vi "GEOM_Adjust_Sizes.vi"(4 "remaining Y":i32, 6 "remainingX":i32, 7 "BinCorrectionType":T7(ring), 8 "Binning":T5={"x"=1, "y"=1} {"y" min=1; "x" min=1}, 9 "sections":T6[](array[typedef]), 10 "Amplifier":T1={"number"=0, "type"=0, "rotated"=0, "fliped"=0, "FPAcoord"={"xstart"=1, "ystart"=1}, "Physical_size"={"columns"=0, "rows"=0}, "predata"={"columns"=0, "rows"=0}, "postdata"={"columns"=0, "rows"=0}, "Req ROIs"=[], "Corr ROI"=[], "Detnumber"=0, "ampID"="", "discard"=0} {"fliped" items=["none", "horizontal", "vertical"]; "type" items=["LL", "LR", "UL", "UR"]}) -> (1 "binned amp":T1={"number"=0, "type"=0, "rotated"=0, "fliped"=0, "FPAcoord"={"xstart"=1, "ystart"=1}, "Physical_size"={"columns"=0, "rows"=0}, "predata"={"columns"=0, "rows"=0}, "postdata"={"columns"=0, "rows"=0}, "Req ROIs"=[], "Corr ROI"=[], "Detnumber"=0, "ampID"="", "discard"=0} {"fliped" items=["none", "horizontal", "vertical"]; "type" items=["LL", "LR", "UL", "UR"]}, 2 "non-binned amp":T1={"number"=0, "type"=0, "rotated"=0, "fliped"=0, "FPAcoord"={"xstart"=1, "ystart"=1}, "Physical_size"={"columns"=0, "rows"=0}, "predata"={"columns"=0, "rows"=0}, "postdata"={"columns"=0, "rows"=0}, "Req ROIs"=[], "Corr ROI"=[], "Detnumber"=0, "ampID"="", "discard"=0} {"fliped" items=["none", "horizontal", "vertical"]; "type" items=["LL", "LR", "UL", "UR"]})   [LabVIEW 2016]
uses:
  GEOM_Moifier.ctl
  GEOM_Amplifier.ctl
  GEOM_AmpType.ctl
  GEOM_ROI.ctl
  GEOM_Coords.ctl
  GEOM_Binning.ctl
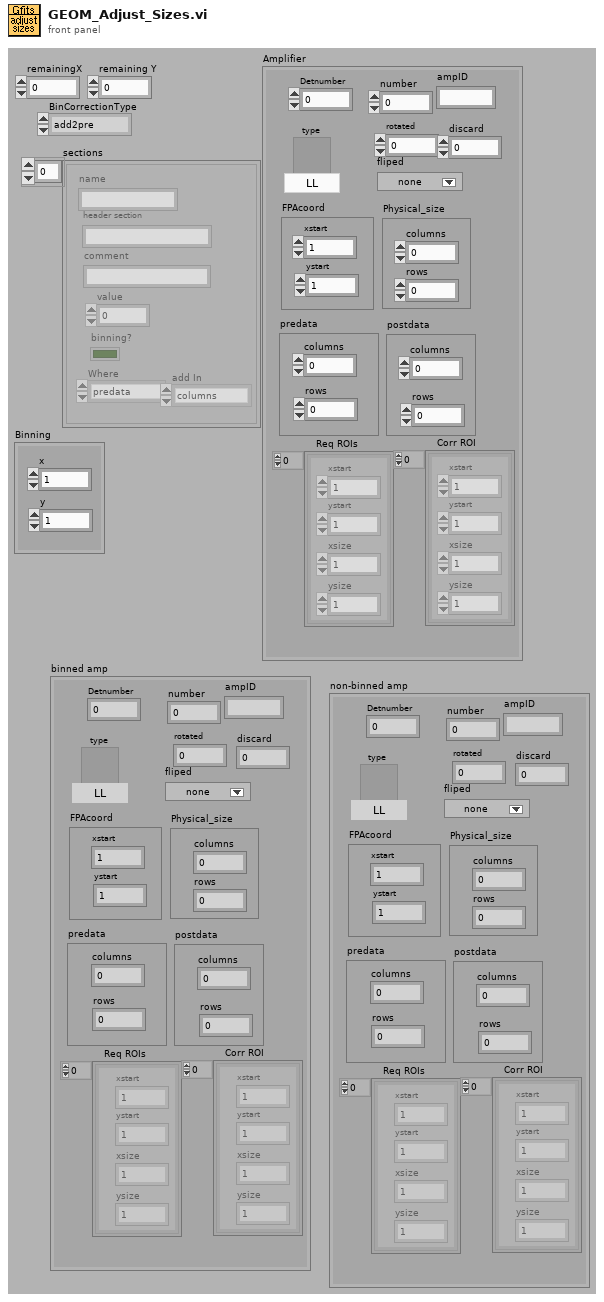
[diagram p1: front panel]
types:
  T1 = typedef "GEOM_Amplifier.ctl" = cluster{"number":i32, "type":T2, "rotated":i16, "fliped":u16, "FPAcoord":cluster{"xstart":i32, "ystart":i32}, "Physical_size":cluster{"columns":i32, "rows":i32}, "predata":cluster{"columns":i32, "rows":i32}, "postdata":cluster{"columns":i32, "rows":i32}, "Req ROIs":T3, "Corr ROI":T3, "Detnumber":i32, "ampID":string, "discard":i32}
  T2 = typedef "GEOM_AmpType.ctl" = u16
  T3 = typedef "GEOM_ROI.ctl" = T4[]
  T4 = typedef "GEOM_Coords.ctl" = cluster{"xstart":u32, "ystart":u32, "xsize":u32, "ysize":u32}
  T5 = typedef "GEOM_Binning.ctl" = cluster{"x":u32, "y":u32}
  T6 = typedef "GEOM_Moifier.ctl" = cluster{"name":string, "header section":string, "comment":string, "value":i32, "binning?":bool, "Where":enum16{"predata", "postdata"}, "add In":enum16{"columns", "rows", "none"}}
  T7 = enum16{"add2pre", "add2post", "add2data", "none"}
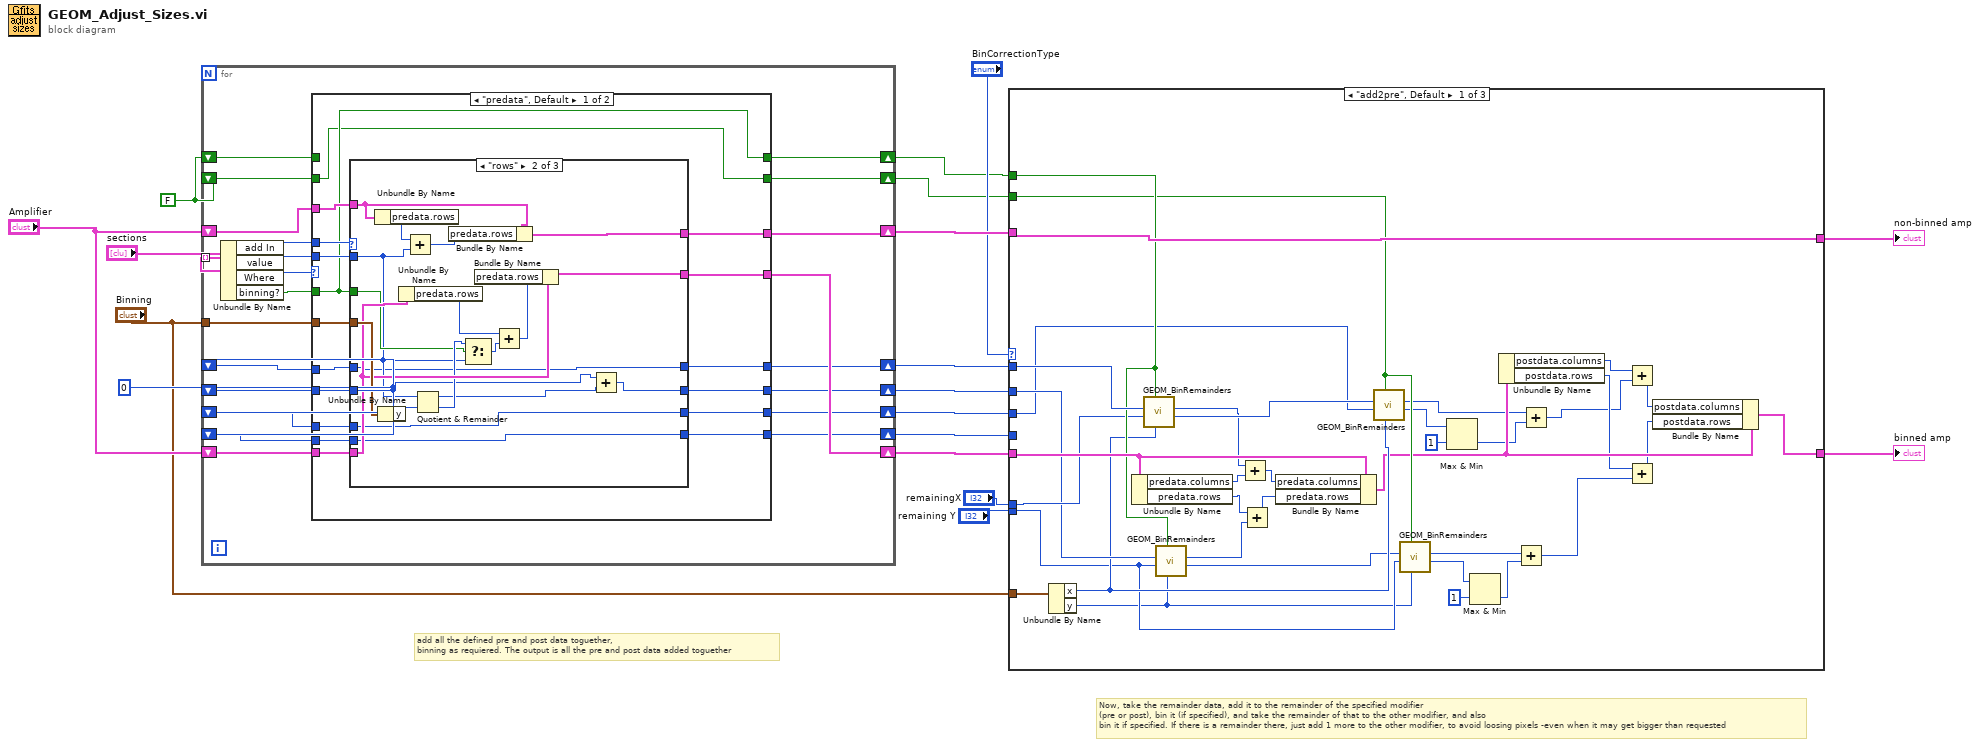
[diagram p0: block diagram]
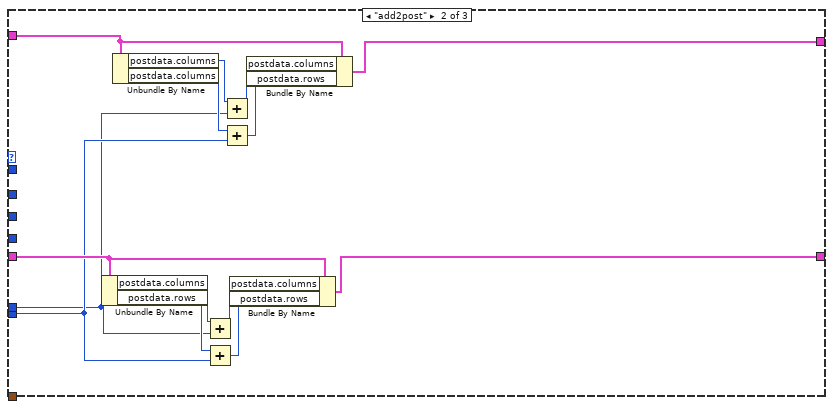
[diagram p2: hidden frame]
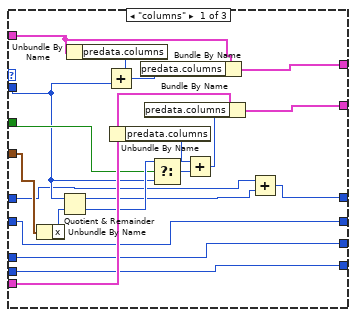
[diagram p4: hidden frame]
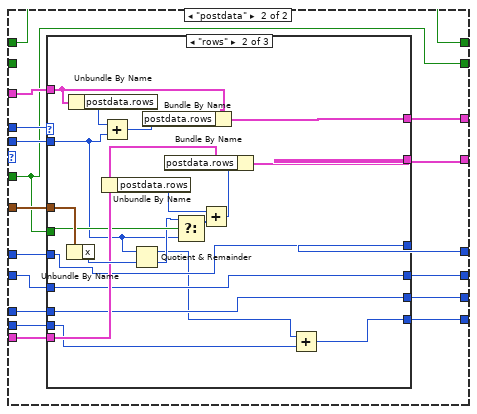
[diagram p6: hidden frame]
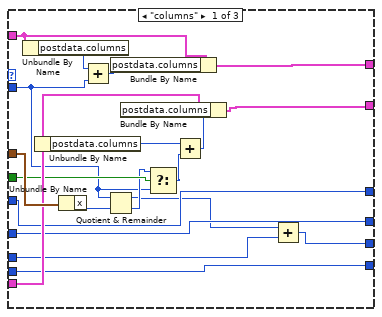
[diagram p7: hidden frame]
diagram:
  w3 = FALSE
  w11 = u32 0
  # "Now, take the remainder data, add it to the remainder of the specified modifier\n(pre or post), bin it (if specified), and take the remainder of that to the other modifier, and also\nbin it if specified. If there is a remainder there, just add 1 more to the other modifier, to avoid loosing pixels -even when it may get bigger than requested"
  # "add all the defined pre and post data toguether,\nbinning as requiered. The output is all the pre and post data added toguether"
  n1 = for {
    tunnel: "sections" -> [w40] mode=indexing
    shift-right: [w36] -> w17
    shift-left: "Amplifier" -> [w31]
    tunnel: "Binning" -> [w34]
    shift-right: [w32] -> w18
    shift-left: "Amplifier" -> [w33]
    shift-right: [w29] -> w15
    shift-left: w11 -> [w30]
    shift-right: [w28] -> w14
    shift-left: w11 -> [w27]
    shift-right: [w26] -> w13
    shift-left: w11 -> [w25]
    shift-right: [w23] -> w12
    shift-left: w11 -> [w24]
    shift-right: [w19] -> w1
    shift-left: w3 -> [w20]
    shift-right: [w22] -> w2
    shift-left: w3 -> [w21]
    n2 = Unbundle By Name(w40) -> ("add In"=w38:enum16{"columns", "rows", "none"}, "value"=w37:i32, "Where"=w39:enum16{"predata", "postdata"}, "binning?"=w35:bool)
    n3 = case shown="\"predata\", Default" w39 {
      tunnel: w38 -> [w57 w120]
      tunnel: w37 -> [w55 w118]
      tunnel: w31 -> [w56 w119]
      tunnel: [w54 w117] -> w36
      tunnel: w35 -> [w42 w105]
      tunnel: w34 -> [w53 w116]
      tunnel: w33 -> [w52 w115]
      tunnel: [w51 w114] -> w32
      tunnel: w30 -> [w50 w111]
      tunnel: [w49 w112] -> w29
      tunnel: [w48 w110] -> w28
      tunnel: w27 -> [w47 w109]
      tunnel: [w46 w113] -> w26
      tunnel: w25 -> [w45 w108]
      tunnel: w24 -> [w44 w106]
      tunnel: [w43 w107] -> w23
      tunnel: [w42 w104] -> w22
      tunnel: w21 -> [_ w104]
      tunnel: w20 -> [w41 _]
      tunnel: [w41 w105] -> w19
      frame "predata", Default {
        n4 = case shown="\"rows\"" w57 {
          tunnel: w56 -> [w71 w95 w103]
          tunnel: w55 -> [w65 w85 _]
          tunnel: [w75 w94 w103] -> w54
          tunnel: w42 -> [w66 w86 _]
          tunnel: w53 -> [w74 w93 _]
          tunnel: w52 -> [w69 w90 w102]
          tunnel: [w68 w89 w102] -> w51
          tunnel: w50 -> [w60 w83 w101]
          tunnel: [w58 w83 w101] -> w49
          tunnel: [w63 w78 w100] -> w48
          tunnel: w47 -> [w63 w80 w100]
          tunnel: [w62 w82 w99] -> w46
          tunnel: w45 -> [w62 w82 w99]
          tunnel: w44 -> [w61 w81 w98]
          tunnel: [w61 w81 w98] -> w43
          frame "columns" {
            n5 = Unbundle By Name(w74) -> ("x"=w73:u32)
            n6 = Quotient & Remainder(x=w65, y=w73) -> (x-y*floor(x/y)=w59:u32, floor(x/y)=w67:u32)
            n7 = Unbundle By Name(w71) -> ("predata.columns"=w76:i32)
            n8 = Add(x=w76, y=w65) -> (x+y=w77:i32)
            n9 = Unbundle By Name(w69) -> ("predata.columns"=w72:i32)
            n10 = Bundle By Name(cluster=w71, "predata.columns"=w77) -> (w75:T1)
            n11 = Select(t=w67, s=w66, f=w65) -> (s? t:f=w64:u32)
            n12 = Add(x=w72, y=w64) -> (x+y=w70:u32)
            n13 = Bundle By Name(cluster=w69, "predata.columns"=w70) -> (w68:T1)
            n14 = Add(x=w60, y=w59) -> (x+y=w58:u32)
          }
          frame "rows" {
            n15 = Unbundle By Name(w95) -> ("predata.rows"=w96:i32)
            n16 = Unbundle By Name(w93) -> ("y"=w91:u32)
            n17 = Unbundle By Name(w90) -> ("predata.rows"=w88:i32)
            n18 = Add(x=w96, y=w85) -> (x+y=w97:i32)
            n19 = Quotient & Remainder(x=w85, y=w91) -> (x-y*floor(x/y)=w79:u32, floor(x/y)=w87:u32)
            n20 = Bundle By Name(cluster=w95, "predata.rows"=w97) -> (w94:T1)
            n21 = Select(t=w87, s=w86, f=w85) -> (s? t:f=w84:u32)
            n22 = Add(x=w88, y=w84) -> (x+y=w92:u32)
            n23 = Bundle By Name(cluster=w90, "predata.rows"=w92) -> (w89:T1)
            n24 = Add(x=w80, y=w79) -> (x+y=w78:u32)
          }
          frame "none", Default {
          }
        }
      }
      frame "postdata" {
        n25 = case shown="\"rows\"" w120 {
          tunnel: w119 -> [w138 w158 w166]
          tunnel: w118 -> [w127 w147 _]
          tunnel: [w137 w157 w166] -> w117
          tunnel: w116 -> [w135 w154 _]
          tunnel: w115 -> [w134 w153 w165]
          tunnel: [w133 w152 w165] -> w114
          tunnel: w105 -> [w132 w151 _]
          tunnel: [w121 w144 w162] -> w113
          tunnel: [w126 w146 w164] -> w112
          tunnel: w111 -> [w126 w146 w164]
          tunnel: [w125 w145 w163] -> w110
          tunnel: w109 -> [w125 w145 w163]
          tunnel: w108 -> [w123 w144 w162]
          tunnel: [w124 w141 w161] -> w107
          tunnel: w106 -> [w124 w143 w161]
          frame "columns" {
            n26 = Unbundle By Name(w138) -> ("postdata.columns"=w139:i32)
            n27 = Unbundle By Name(w134) -> ("postdata.columns"=w130:i32)
            n28 = Unbundle By Name(w135) -> ("x"=w136:u32)
            n29 = Add(x=w139, y=w127) -> (x+y=w140:i32)
            n30 = Quotient & Remainder(x=w127, y=w136) -> (x-y*floor(x/y)=w122:u32, floor(x/y)=w129:u32)
            n31 = Bundle By Name(cluster=w138, "postdata.columns"=w140) -> (w137:T1)
            n32 = Select(t=w129, s=w132, f=w127) -> (s? t:f=w131:u32)
            n33 = Add(x=w130, y=w131) -> (x+y=w128:u32)
            n34 = Bundle By Name(cluster=w134, "postdata.columns"=w128) -> (w133:T1)
            n35 = Add(x=w122, y=w123) -> (x+y=w121:u32)
          }
          frame "rows" {
            n36 = Unbundle By Name(w154) -> ("x"=w156:u32)
            n37 = Unbundle By Name(w158) -> ("postdata.rows"=w159:i32)
            n38 = Add(x=w159, y=w147) -> (x+y=w160:i32)
            n39 = Unbundle By Name(w153) -> ("postdata.rows"=w148:i32)
            n40 = Quotient & Remainder(x=w147, y=w156) -> (x-y*floor(x/y)=w142:u32, floor(x/y)=w150:u32)
            n41 = Bundle By Name(cluster=w158, "postdata.rows"=w160) -> (w157:T1)
            n42 = Select(t=w150, s=w151, f=w147) -> (s? t:f=w149:u32)
            n43 = Add(x=w148, y=w149) -> (x+y=w155:u32)
            n44 = Bundle By Name(cluster=w153, "postdata.rows"=w155) -> (w152:T1)
            n45 = Add(x=w142, y=w143) -> (x+y=w141:u32)
          }
          frame "none", Default {
          }
        }
      }
    }
  }
  n46 = case shown="\"add2pre\", Default" "BinCorrectionType" {
    tunnel: [w196 w212 w217] -> w6
    tunnel: w18 -> [w202 w211 w217]
    tunnel: w17 -> [w200 w206 w218]
    tunnel: [w200 w205 w218] -> w7
    tunnel: "remaining Y" -> [w190 w204 _]
    tunnel: "remainingX" -> [w197 w203 _]
    tunnel: w15 -> [w199 _ _]
    tunnel: w14 -> [w195 _ _]
    tunnel: w13 -> [w193 _ _]
    tunnel: w12 -> [_ _ _]
    tunnel: "Binning" -> [w201 _ _]
    tunnel: w2 -> [w198 _ _]
    tunnel: w1 -> [w188 _ _]
    frame "add2pre", Default {
      n47 = Unbundle By Name(w201) -> ("x"=w192:u32, "y"=w189:u32)
      n48 = Unbundle By Name(w202) -> ("predata.columns"=w186:i32, "predata.rows"=w183:i32)
      n49 = call "GEOM_BinRemainders.vi"("bin factor"=w192, "bin?"=w198, "remaining data"=w197, "remaining modif"=w199) -> ("remaining remainder"=w194:i32, "out value"=w187:i32)  [unwired: 6 out]
      n50 = call "GEOM_BinRemainders.vi"("bin factor"=w189, "bin?"=w198, "remaining data"=w190, "remaining modif"=w195) -> ("remaining remainder"=w191:i32, "out value"=w184:i32)  [unwired: 6 out]
      n51 = Add(x=w187, y=w186) -> (x+y=w185:i32)
      n52 = Add(x=w183, y=w184) -> (x+y=w182:i32)
      n53 = Bundle By Name(cluster=w202, "predata.columns"=w185, "predata.rows"=w182) -> (w181:T1)
      n54 = call "GEOM_BinRemainders.vi"("bin factor"=w192, "bin?"=w188, "remaining data"=w193, "remaining modif"=w194) -> ("remaining remainder"=w172:i32, "out value"=w176:i32)  [unwired: 6 out]
      n55 = call "GEOM_BinRemainders.vi"("bin factor"=w189, "bin?"=w188, "remaining data"=w190, "remaining modif"=w191) -> ("remaining remainder"=w168:i32, "out value"=w174:i32)  [unwired: 6 out]
      n56 = Max & Min(x=w172, y=1) -> (min(x,y)=w170:i32)  [unwired: 1 out]
      n57 = Max & Min(x=w168, y=1) -> (min(x,y)=w167:i32)  [unwired: 1 out]
      n58 = Unbundle By Name(w181) -> ("postdata.columns"=w178:i32, "postdata.rows"=w180:i32)
      n59 = Add(x=w174, y=w167) -> (x+y=w173:i32)
      n60 = Add(x=w176, y=w170) -> (x+y=w175:i32)
      n61 = Add(x=w178, y=w175) -> (x+y=w177:i32)
      n62 = Add(x=w180, y=w173) -> (x+y=w179:i32)
      n63 = Bundle By Name(cluster=w181, "postdata.columns"=w177, "postdata.rows"=w179) -> (w196:T1)
    }
    frame "add2post" {
      n64 = Unbundle By Name(w211) -> ("postdata.columns"=w216:i32, "postdata.rows"=w215:i32)
      n65 = Unbundle By Name(w206) -> ("postdata.columns"=w210:i32, "postdata.columns"=w209:i32)
      n66 = Add(x=w216, y=w203) -> (x+y=w214:i32)
      n67 = Add(x=w215, y=w204) -> (x+y=w213:i32)
      n68 = Add(x=w210, y=w203) -> (x+y=w208:i32)
      n69 = Add(x=w209, y=w204) -> (x+y=w207:i32)
      n70 = Bundle By Name(cluster=w211, "postdata.columns"=w214, "postdata.rows"=w213) -> (w212:T1)
      n71 = Bundle By Name(cluster=w206, "postdata.columns"=w208, "postdata.rows"=w207) -> (w205:T1)
    }
    frame "none" {
    }
  }
  "non-binned amp" <- w7
  "binned amp" <- w6
